vi "Build_Plot_Selection-Acquire.vi"(5 "Audio Device Details":T3(array[cluster]), 7 "Audio Settings":T1, 8 "error in (no error)":errorcluster) -> (0 "error out":errorcluster, 3 "Plot Selection":T2(array[cluster]))   [LabVIEW 2020]
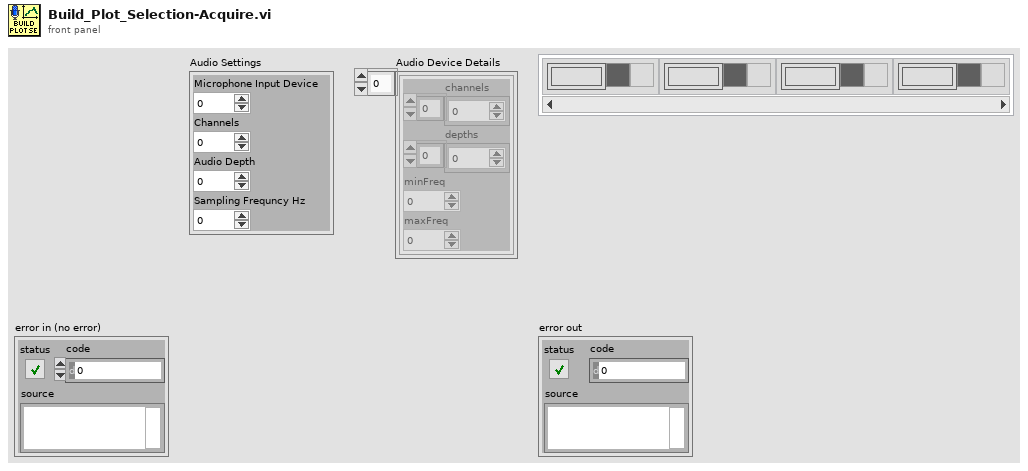
[diagram p1: front panel]
types:
  T1 = cluster{"Microphone Input Device":u32, "Channels":i32, "Audio Depth":i32, "Sampling Frequncy Hz":dbl}
  T2 = cluster{"Plot Name":string, "Plot Color":u32, "Visibility":bool}[]
  T3 = cluster{"channels":i32[], "depths":i32[], "minFreq":dbl, "maxFreq":dbl}[]
  T4 = cluster{"Plot Name":string, "Plot Color":u32, "Visibility":bool}
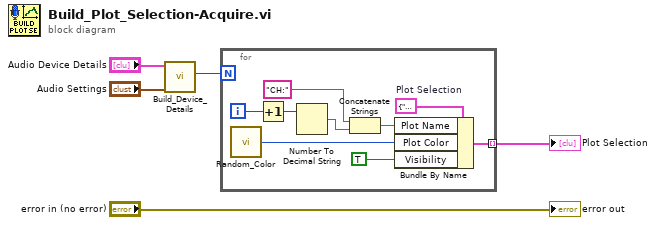
[diagram p0: block diagram]
diagram:
  n1 = call "Build_Device_Details.vi"("Audio Settings"="Audio Settings", "Audio Device Details"="Audio Device Details") -> ("Channel"=w2:i32)  [unwired: 4 in, 5 out]
  n2 = for {
    N: w2 -> [_]
    tunnel: [w13] -> w5 mode=indexing
    i -> [w11]
    w14 = T4 {"Plot Name"="", "Plot Color"=0, "Visibility"=FALSE}  # Plot Selection
    n3 = call "Random_Color.vi"() -> ("Color"=w12:u32)
    n4 = Increment(x=w11) -> (x+1=w7:i32)
    n5 = Number To Decimal String(number=w7) -> (decimal integer string=w6:string)  [unwired: 1 in]
    n6 = Concatenate Strings("CH:", w6) -> (w9:string)
    n7 = Bundle By Name(cluster=w14, "Plot Name"=w9, "Plot Color"=w12, "Visibility"=TRUE) -> (w13:T4)
  }
  "Plot Selection" <- w5
  "error out" <- "error in (no error)"
